vi "check_done(第二站).vi"(10 "Boolean":bool) -> (2 "Release Queue":T1[](array[typedef]))   [LabVIEW 2016]
uses:
  Message Queue/Message Cluster.ctl
  Message Queue/Message Queue.lvlib
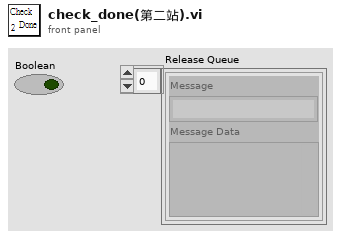
[diagram p1: front panel]
types:
  T1 = typedef "Message Queue.lvlib/Message Cluster.ctl" = cluster{"Message":string, "Message Data":variant}
  T2 = enum16{"Open", "Enqueue", "InsertQueue", "Release Queue", "Close"}
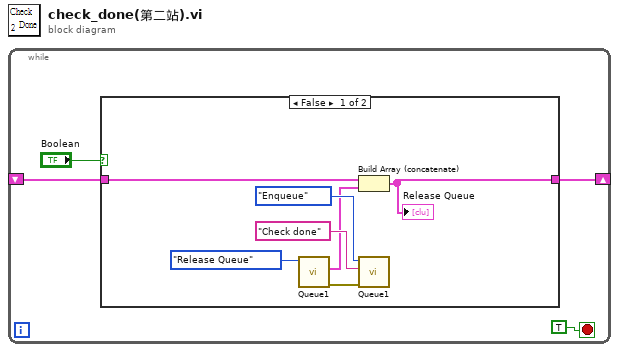
[diagram p0: block diagram]
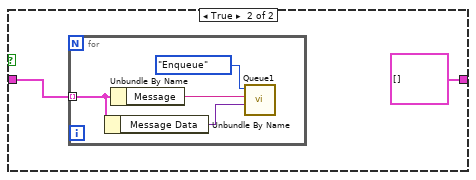
[diagram p2: hidden frame]
diagram:
  n1 = while {
    shift-right: [w1] -> _
    shift-left: _ -> [w2]
    stop <- TRUE stop-if-true
    n2 = case shown="False" "Boolean" {
      tunnel: w2 -> [w7 w12]
      tunnel: [w5 T1[] [] ("Release Queue")] -> w1
      frame False {
        n3 = call "Queue1.vi"("Function"=T2."Release Queue") -> ("error out"=w8:errorcluster, "Release Queue"=w6:T1[])  [unwired: 8 in, 1 out]
        n4 = Build Array (concatenate)(w7, w6) -> (w5:T1[])
        "Release Queue" <- w5
        n5 = call "Queue1.vi"("error in"=w8, "Message"="Check done", "Function"=T2."Enqueue") -> ()  [unwired: 6 in, 3 out]
      }
      frame True {
        n6 = for {
          tunnel: w12 -> [w15] mode=indexing
          n7 = Unbundle By Name(w15) -> ("Message Data"=w14:variant)
          n8 = Unbundle By Name(w15) -> ("Message"=w16:string)
          n9 = call "Queue1.vi"("Message Data"=w14, "Message"=w16, "Function"=T2."Enqueue") -> ()  [unwired: 6 in, 3 out]
        }
      }
    }
  }
